vi "MessageHandling.vi"(8 "Reply":string, 9 "Message":T1={"Recv ["="msg_start\n", "Recv ]"="msg_end", "Reply ["="reply_start\n", "Reply ]"="reply_end"}, 11 "REPL":string) -> (0 "New Reply":string, 1 "New Message":string, 2 "New Message?":bool=TRUE, 3 "# done msg":i32)   [LabVIEW 2020]
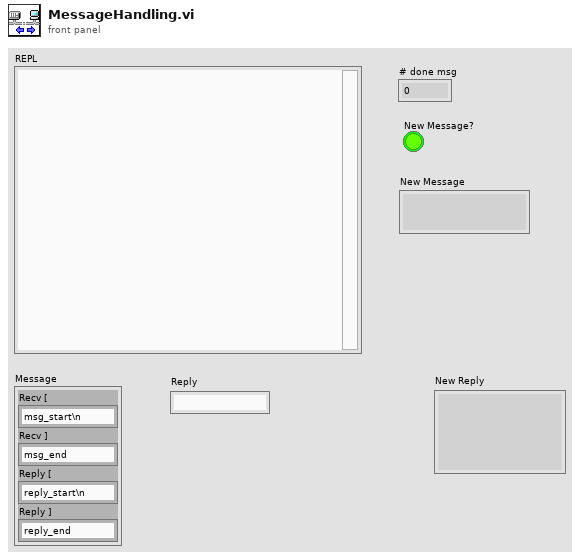
[diagram p1: front panel]
types:
  T1 = cluster{"Recv [":string, "Recv ]":string, "Reply [":string, "Reply ]":string}
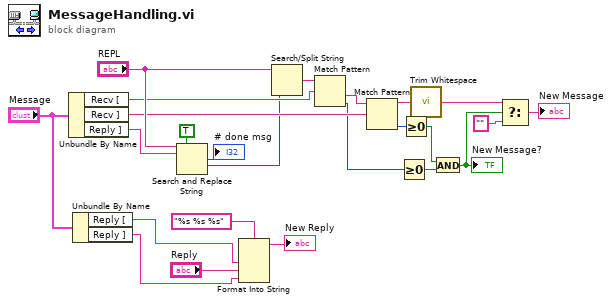
[diagram p0: block diagram]
diagram:
  n1 = Unbundle By Name("Message") -> ("Recv ["=w19:string, "Recv ]"=w17:string, "Reply ]"=w24:string)
  n2 = Unbundle By Name("Message") -> ("Reply ["=w5:string, "Reply ]"=w4:string)
  n3 = Search and Replace String(replace all?=TRUE ("replace all? (F)"), input string="REPL", search string=w24) -> (number of replacements=→"# done msg":i32, offset past replacement=w1:i32)  [unwired: 5 in, 2 out]
  n4 = Format Into String(format string="%s %s %s", w5, "Reply", w4) -> (resulting string=→"New Reply":string)  [unwired: 2 in, 1 out]
  n5 = Search/Split String(string="REPL", offset (0)=w1) -> (match + rest of string=w20:string)  [unwired: 1 in, 2 out]
  n6 = Match Pattern(string=w20, regular expression=w19) -> (after substring=w18:string, offset past match=w16:i32)  [unwired: 1 in, 2 out]
  n7 = Match Pattern(string=w18, regular expression=w17) -> (before substring=w11:string, offset past match=w15:i32)  [unwired: 1 in, 2 out]
  n8 = Greater Or Equal To 0?(x=w16) -> (x >= 0?=w13:bool)
  n9 = Greater Or Equal To 0?(x=w15) -> (x >= 0?=w14:bool)
  n10 = call <vilib>:"Trim Whitespace.vi"("string"=w11) -> ("trimmed string"=w2:string)  [unwired: 1 in]
  n11 = And(x=w14, y=w13) -> (x .and. y?=w12:bool)
  "New Message?" <- w12
  n12 = Select(t=w2, s=w12, f="") -> (s? t:f=→"New Message":string)
